vi "LaunchProcess.vi"(11 "SMO Reference":refnum<class "SMO.lvclass">) -> ()   [LabVIEW 2013, in "SMO.lvclass"]
doc: "Launches the Process VIs.\n\n---------------------------------------------------------------\nJKI State Machine Objects™\nhttp://jki.net/state-machine-objects/\nCopyright (C) 2005-2015, JKI <info@jki.net>\nALL RIGHTS RESERVED"
uses:
  SMO.lvclass
panel:
  # "For instructions on how to use the JKI State Machine Objects, examples and video tutorials, visit:\nhttp://jki.net/state-machine-objects/\n\nJKI State Machine Objects™\nhttp://jki.net/state-machine-objects/\nCopyright (C) 2005-2015, JKI <info@jki.net>\nALL RIGHTS RESERVED"
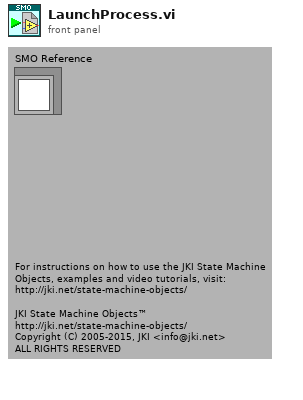
[diagram p1: front panel]
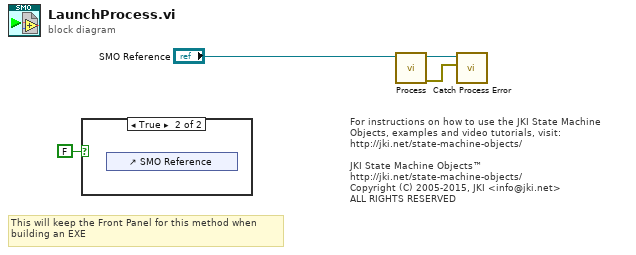
[diagram p0: block diagram]
diagram:
  # "This will keep the Front Panel for this method when\nbuilding an EXE"
  # "For instructions on how to use the JKI State Machine Objects, examples and video tutorials, visit:\nhttp://jki.net/state-machine-objects/\n\nJKI State Machine Objects™\nhttp://jki.net/state-machine-objects/\nCopyright (C) 2005-2015, JKI <info@jki.net>\nALL RIGHTS RESERVED"
  n1 = case shown="True" FALSE {
    frame False {
    }
    frame True {
      n2 = control-ref of="SMO Reference"() -> ()  [unwired: 1 out]
    }
  }
  n3 = call-dynamic "Process.vi"("SMO"="SMO Reference") -> ("error out"=w2:errorcluster, "SMO out"=w3:refnum<class "SMO.lvclass">)  [unwired: 9 in]
  n4 = call "Catch Process Error.vi"("Process Error"=w2, "SMO"=w3) -> ()  [unwired: 10 in]
